vi "SetDAC.vi"(8 "error in":T1, 10 "Value [V]":T2=-inf format="%#_g V", 11 "Number":T3 items=["DAC 1", "DAC 2", "DAC 3", "DAC 4"]) -> (0 "error out":T1, 2 "Value":sgl format="%#_g V", 3 "Number out":i32)   [LabVIEW 2016]
doc: "The DAC addressed by 'number', which is a required input [0 to 3], is set to the 'value'. The value has to be given in V and is generally restricted from -10V to +10V. In addition the value cannot exceed the set DAC limits which can be set with the setDACLimits.vi."
uses:
  Controls/DAC_Selection.ctl
  Controls/DAC_Voltage.ctl
  Controls/Error_Out.ctl
  Files_ASC500/DLL/ASC500_RemoteControlV27.dll
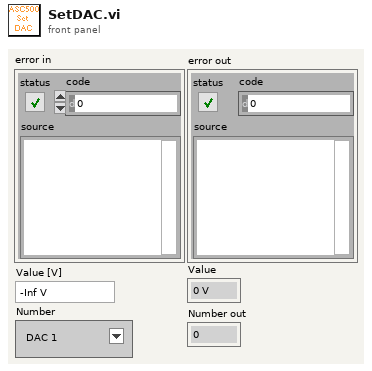
[diagram p1: front panel]
types:
  T1 = typedef "Error_Out.ctl" = errorcluster
  T2 = typedef "DAC_Voltage.ctl" = sgl
  T3 = typedef "DAC_Selection.ctl" = u16
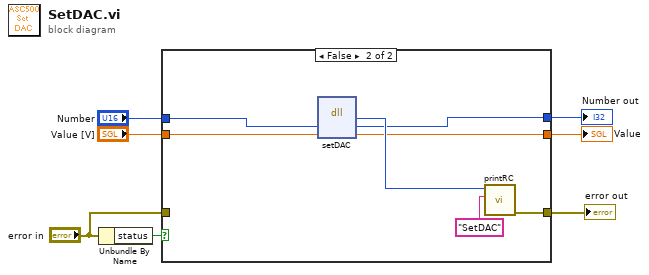
[diagram p0: block diagram]
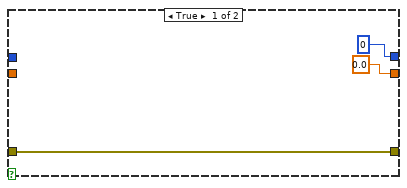
[diagram p2: hidden frame]
diagram:
  n1 = Unbundle By Name("error in") -> ("status"=w7:bool)
  n2 = case shown="False" w7 {
    tunnel: [w10 w15] -> w6
    tunnel: "Number" -> [_ w17]
    tunnel: "Value [V]" -> [_ w16]
    tunnel: "error in" -> [w10 _]
    tunnel: [0 ("Number") w12] -> w2
    tunnel: [sgl 0.0 ("Value") w11] -> w1
    frame True {
    }
    frame False {
      n3 = dll-call lib="G:/SCMOperations/Share/ELE/Produkt Information/ASC500/04 Remote Control/02 development versions/2018Nov06/Files_ASC500/DLL/ASC500_RemoteControlV27.dll" fn="setDAC"("Number"=w17, "Value"=w16) -> ("return type"=w14:i32, "Number"=w12:i32, "Value"=w11:sgl)  [unwired: 3 in, 2 out]
      n4 = call "printRC.vi"("additional information"="SetDAC", "RC"=w14) -> ("error out"=w15:T1)  [unwired: 9 in]
    }
  }
  "error out" <- w6
  "Number out" <- w2
  "Value" <- w1
